vi "MDF_Set_Default_Install.vi"(8 "error in (no error)":errorcluster, 11 "absFolder in":refnum<class "absFolder.lvclass">) -> (0 "error out":errorcluster)   [LabVIEW 2020, in "absFolder.lvclass"]
uses:
  <vilib>/AppBuilder/IB_Classes/Destination/absFolder/absFolder.lvclass
  <vilib>/AppBuilder/IB_Classes/Destination/absFolder/absFolder.lvclass/absFolder.ctl
  AppLibs/distkit/MDF/NIMdf.llb/MDFBDPAddFilePathType.ctl
  AppLibs/distkit/MDF/NI_MDF.lvlib
  <vilib>/AppBuilder/IB_Classes/Destination/IB_Destination.lvclass
  AppLibs/distkit/MDF/NIMdf.llb/MDFBuildDevPart_SetDefaultInstallDir (string).vi
  e:/builds/penguin/labview/branches/2020/dev/dist/vi.lib/AppBuilder/IB_Classes/Destination/IB_Destination.lvclass
  e:/builds/penguin/labview/branches/2020/dev/dist/vi.lib/AppBuilder/IB_Classes/Destination/absFolder/absFolder.lvclass
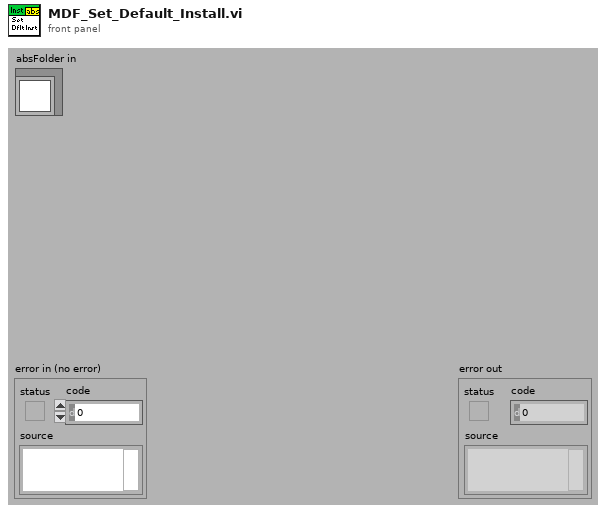
[diagram p1: front panel]
types:
  T1 = typedef "NI_MDF.lvlib/MDFBDPAddFilePathType.ctl" = i32
  T2 = typedef "IB_Destination.ctl" = cluster{"name":string, "unlock":bool, "parentTag":string, "destTag":string, "eng_installPath":string}
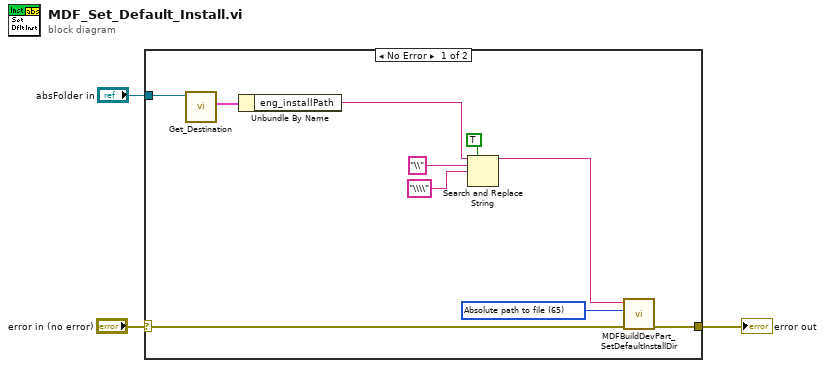
[diagram p0: block diagram]
diagram:
  n1 = case shown="No Error" "error in (no error)" {
    selector: "error in (no error)" -> [w12 w14]
    tunnel: [w11 w14] -> w1
    tunnel: "absFolder in" -> [w10 _]
    frame No Error {
      w13 = T1 65 items=["Relative to default installation directory"=68, "Root directory on first partition"=70, "Relative to directory table key"=82, "Absolute path to file"=65] ("installation directory path type (Root directory on first partition)")
      n2 = call <vilib>:"Get_Destination.vi"("IB_Destination in"=w10) -> ("data"=w9:T2)  [unwired: 1 in, 9 out]
      n3 = Unbundle By Name(w9) -> ("eng_installPath"=w7:string)
      n4 = Search and Replace String(replace all?=TRUE ("replace all? (F)"), input string=w7, search string="\\", replace string="\\\\" ("replace string (\"\")")) -> (result string=w8:string)  [unwired: 4 in, 3 out]
      n5 = call-poly "MDFBuildDevPart_SetDefaultInstallDir.vi"("error in (no error)"=w12, "installation directory path type (Root directory on first partition)"=w13, "default installation directory"=w8) -> ("error out"=w11:errorcluster)  [unwired: 8 in]
    }
    frame Error {
    }
  }
  "error out" <- w1
